vi "XY Graph Merge Selected Plots Event.vi"(8 "Error In":errorcluster, 9 "Merge All Plots? (T)":bool=TRUE, 11 "XYGraph Ref":T1) -> (0 "Error Out":errorcluster, 1 "Message":string)   [LabVIEW 2021, in "XY Graph Add-Ons.lvlib"]
uses:
  XY Graph Add-Ons.lvlib
  XY Graph Refnum.ctl
  XY Plot Data.ctl
  XY Graph Add Single Plot with Name.vi
  Strings/Strings.lvlib
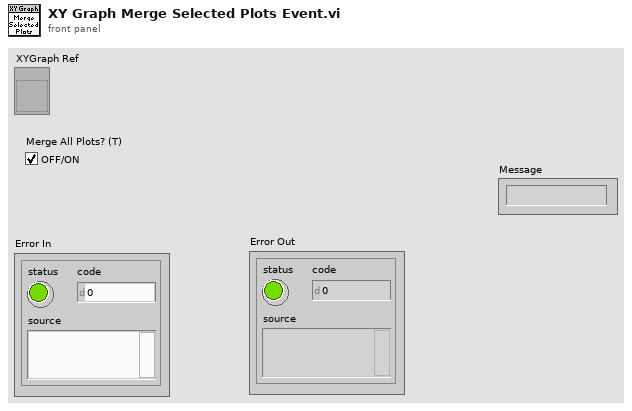
[diagram p1: front panel]
types:
  T1 = typedef "XY Graph Add-Ons.lvlib/XY Graph Refnum.ctl" = refnum<vi>
  T2 = typedef "XY Graph Add-Ons.lvlib/XY Plot Data.ctl" = cluster{"X Array":dbl[], "Y Array":dbl[]}
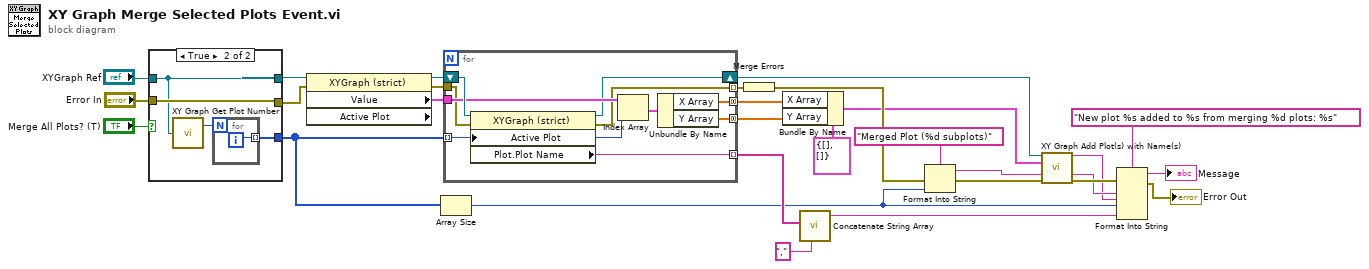
[diagram p0: block diagram]
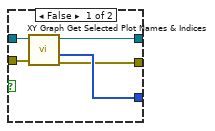
[diagram p2: hidden frame]
diagram:
  n1 = case shown="True" "Merge All Plots? (T)" {
    tunnel: "XYGraph Ref" -> [w34 w37]
    tunnel: "Error In" -> [w33 w38]
    tunnel: [w32 w37] -> w27
    tunnel: [w31 w35] -> w16
    tunnel: [w30 w38] -> w26
    frame False {
      n2 = call "XY Graph Get Selected Plot Names & Indices.vi"("error in (no error)"=w33, "XYGraph in"=w34) -> ("error out"=w30:errorcluster, "Selected Plots"=w31:i32[], "XYGraph out"=w32:T1)  [unwired: 5 in, 2 out]
    }
    frame True {
      n3 = call "XY Graph Get Plot Number.vi"("XYGraph"=w37) -> ("# Plots"=w36:i32)  [unwired: 8 in]
      n4 = for {
        N: w36 -> [_]
        tunnel: [w39] -> w35 mode=indexing
        i -> [w39]
      }
    }
  }
  n5 = property class="XYGraph (strict)" props=["Value", "Active Plot"](reference=w27, error in=w26) -> (reference out=w24:T1, error out=w23:errorcluster, "Value"=w18:cluster{"X Array":dbl[], "Y Array":dbl[]}[])  [unwired: 1 out]
  n6 = Array Size(array=w16) -> (size(s)=w4:i32)
  n7 = for {
    tunnel: w16 -> [w46] mode=indexing
    tunnel: [w48] -> w14 mode=indexing
    tunnel: w18 -> [w47]
    tunnel: [w44] -> w21 mode=concatenating
    tunnel: [w43] -> w20 mode=concatenating
    shift-right: [w42] -> w12
    shift-left: w24 -> [w49]
    tunnel: w23 -> [w41]
    tunnel: [w40] -> w22 mode=indexing
    n8 = property class="XYGraph (strict)"(reference=w49, error in=w41, "Active Plot"=w46) -> (reference out=w42:T1, error out=w40:errorcluster, "Plot.Plot Name"=w48:string)
    n9 = Index Array(array=w47, index=w46) -> (element=w45:cluster{"X Array":dbl[], "Y Array":dbl[]})
    n10 = Unbundle By Name(w45) -> ("X Array"=w44:dbl[], "Y Array"=w43:dbl[])
  }
  n11 = Merge Errors(w22) -> (w15:errorcluster)
  n12 = Bundle By Name(cluster=T2 {"X Array"=[], "Y Array"=[]} ("input cluster"), "X Array"=w21, "Y Array"=w20) -> (w11:T2)
  n13 = call "Concatenate String Array.vi"("Separator (TAB)"=",", "String Array"=w14) -> ("Formatted String"=w3:string)  [unwired: 9 in]
  n14 = Format Into String(format string="Merged Plot (%d subplots)" ("Plot.Plot Name"), error in=w15, w4) -> (resulting string=w10:string, error out=w9:errorcluster)  [unwired: 1 in]
  n15 = call-poly "XY Graph Add Plot(s) with Name(s).vi"("XYGraph Ref in"=w12, "Plot"=w11, "Plot Name (\"Plot\")"=w10, "error in (no error)"=w9) -> ("XY Graph Caption (or Label)"=w5:string, "Plot Name"=w6:string, "error out"=w8:errorcluster)  [unwired: 8 in, 1 out]
  n16 = Format Into String(format string="New plot %s added to %s from merging %d plots: %s", error in=w8, w6, w5, w4, w3) -> (resulting string=→"Message":string, error out=→"Error Out":errorcluster)  [unwired: 1 in]
